vi "Administrators.vi"(11 "数组":string[](array[string])) -> (1 "成功":bool, 2 "子字符串之后":string, 3 "数组 2":string[](array[string]))   [LabVIEW 2018]
panel:
  in  "权限：":string(combo)
  in  "停止":bool
  in  "按钮":bool
  in  "密码：":string
  in  "用户名：":string
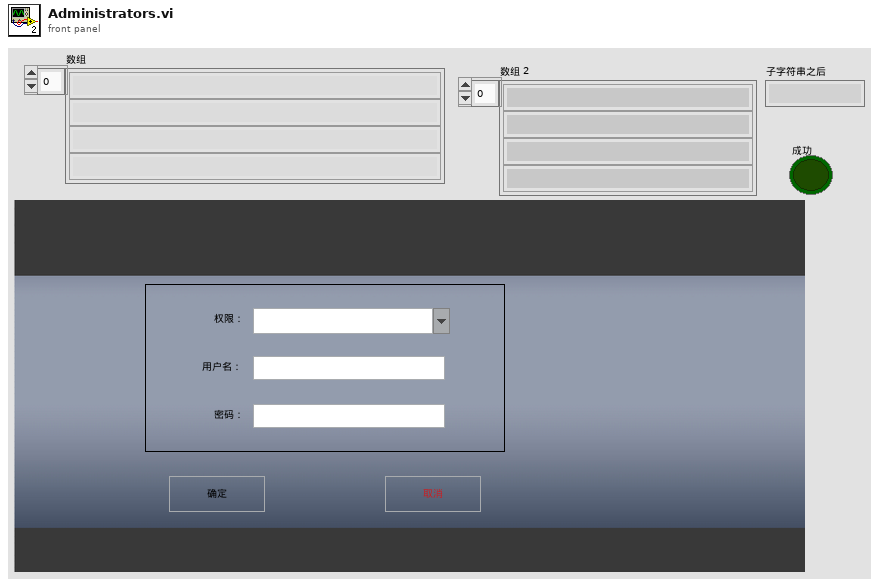
[diagram p1: front panel]
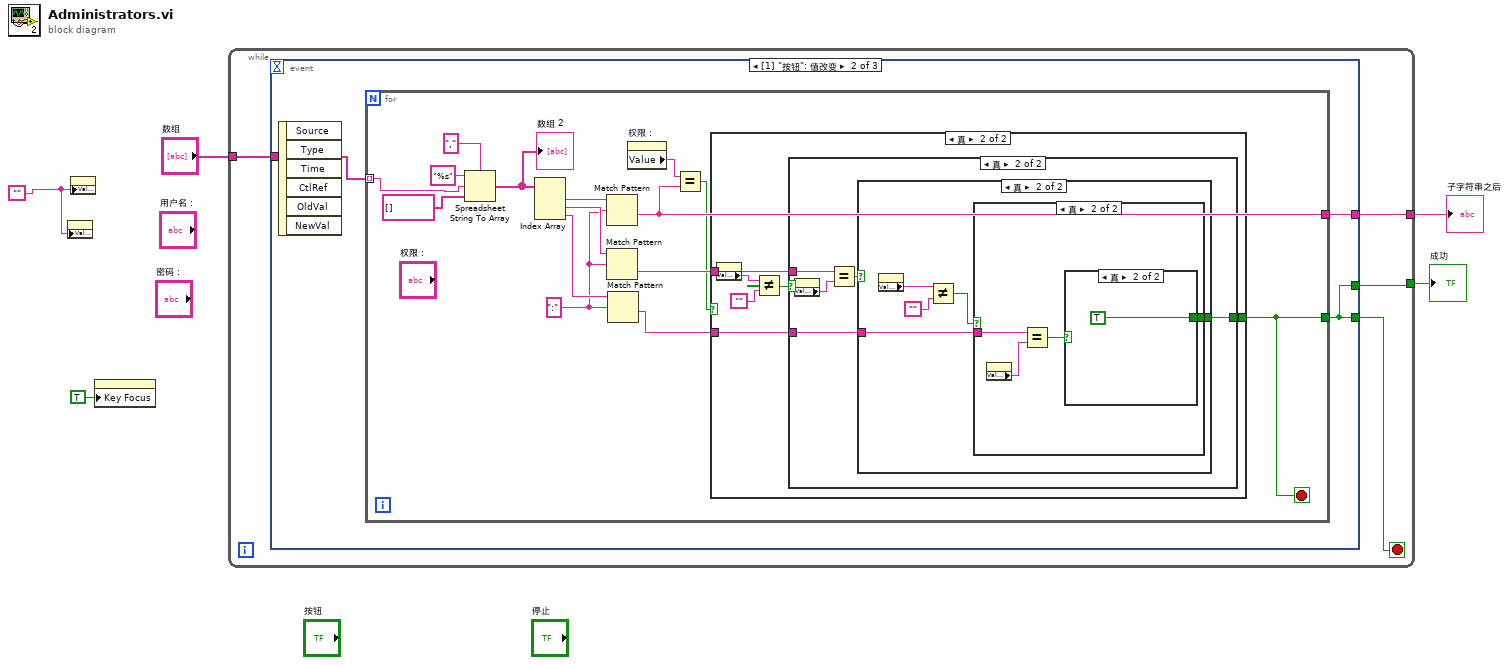
[diagram p0: block diagram]
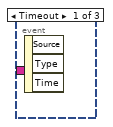
[diagram p2: hidden frame]
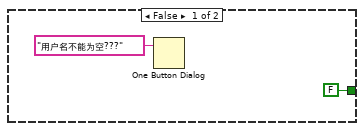
[diagram p4: hidden frame]
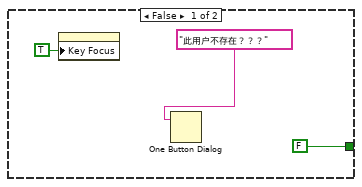
[diagram p5: hidden frame]
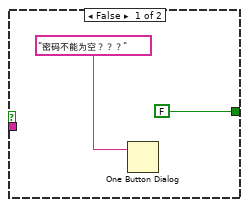
[diagram p6: hidden frame]
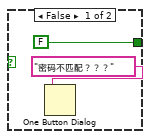
[diagram p7: hidden frame]
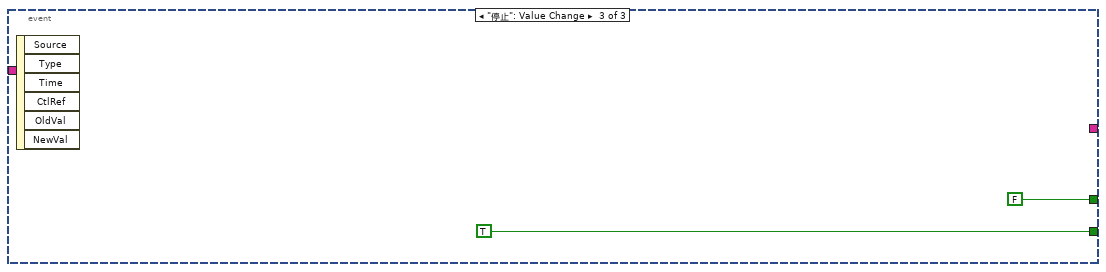
[diagram p8: hidden frame]
diagram:
  w2 = ""
  n1 = property on="密码：" class="Str"("Value"=w2) -> ()  [unwired: 2 in, 2 out]
  n2 = property on="用户名：" class="Str"("Value"=w2) -> ()  [unwired: 2 in, 2 out]
  n3 = property on="用户名：" class="Str"("Key Focus"=TRUE ("键选中")) -> ()  [unwired: 2 in, 2 out]
  n4 = while {
    tunnel: "数组" -> [w9]
    tunnel: [w8] -> w4
    tunnel: [w6] -> w1
    stop <- w7 stop-if-true
    n5 = event shown="[1] \"按钮\": 值改变" {
      selector: _ -> [_ _ _]
      dyn-events: _ -> [_ _ _]
      timeout: _ -> [_ _ _]
      tunnel: w9 -> [_ w12 _]
      tunnel: [_ w10 TRUE] -> w7
      tunnel: [_ w11 _] -> w8
      tunnel: [_ w10 FALSE] -> w6
      event Timeout {
        n6 = event-data() -> ()  [unwired: 1 in, 3 out]
      }
      event "按钮": Value Change {
        n7 = event-data() -> ()  [unwired: 1 in, 6 out]
        n8 = for {
          tunnel: w12 -> [w24] mode=indexing
          tunnel: [w15] -> w11
          tunnel: [w13] -> w10
          stop <- w13 stop-if-true
          w19 = ":" ("正则表达式")
          n9 = Spreadsheet String To Array(delimiter (Tab)="," ("分隔符(Tab)"), format string="%s" ("格式字符串"), spreadsheet string=w24, array type (2D Dbl)=string[] []) -> (array=w23:string[])
          "数组 2" <- w23
          n10 = Index Array(array=w23) -> (element #1=w22:string, element #2=w21:string, element #3=w20:string)  [unwired: 3 in]
          n11 = Match Pattern(string=w22, regular expression=w19) -> (after substring=w15:string)  [unwired: 1 in, 3 out]
          n12 = Match Pattern(string=w21, regular expression=w19) -> (after substring=w18:string)  [unwired: 1 in, 3 out]
          n13 = Match Pattern(string=w20, regular expression=w19) -> (after substring=w17:string)  [unwired: 1 in, 3 out]
          n14 = property on="权限：" class="CmbBox"() -> ("Value"=w16:string)  [unwired: 2 in, 2 out]
          n15 = Equal?(x=w16, y=w15) -> (x = y?=w14:bool)
          n16 = case shown="真" w14 {
            tunnel: w18 -> [_ w32]
            tunnel: w17 -> [_ w30]
            tunnel: [_ w29] -> w13
            frame False {
            }
            frame True {
              n17 = property on="用户名：" class="Str"() -> ("Value"=w28:string)  [unwired: 2 in, 2 out]
              n18 = Not Equal?(x=w28, y="") -> (x != y?=w31:bool)
              n19 = case shown="真" w31 {
                tunnel: w32 -> [_ w38]
                tunnel: w30 -> [_ w37]
                tunnel: [FALSE w36] -> w29
                frame False {
                  n20 = One Button Dialog(message="用户名不能为空???" ("消息")) -> ()  [unwired: 1 in, 1 out]
                }
                frame True {
                  n21 = property on="用户名：" class="Str"() -> ("Value"=w40:string)  [unwired: 2 in, 2 out]
                  n22 = Equal?(x=w38, y=w40) -> (x = y?=w39:bool)
                  n23 = case shown="真" w39 {
                    tunnel: w37 -> [_ w47]
                    tunnel: [FALSE w45] -> w36
                    frame False {
                      n24 = property on="用户名：" class="Str"("Key Focus"=TRUE ("键选中")) -> ()  [unwired: 2 in, 2 out]
                      n25 = One Button Dialog(message="此用户不存在？？？") -> ()  [unwired: 1 in, 1 out]
                    }
                    frame True {
                      n26 = property on="密码：" class="Str"() -> ("Value"=w44:string)  [unwired: 2 in, 2 out]
                      n27 = Not Equal?(x=w44, y="") -> (x != y?=w46:bool)
                      n28 = case shown="真" w46 {
                        tunnel: w47 -> [_ w54]
                        tunnel: [FALSE w51] -> w45
                        frame False {
                          n29 = One Button Dialog(message="密码不能为空？？？") -> ()  [unwired: 1 in, 1 out]
                        }
                        frame True {
                          n30 = property on="密码：" class="Str"() -> ("Value"=w53:string)  [unwired: 2 in, 2 out]
                          n31 = Equal?(x=w54, y=w53) -> (x = y?=w52:bool)
                          n32 = case shown="真" w52 {
                            tunnel: [FALSE TRUE] -> w51
                            frame False {
                              n33 = One Button Dialog(message="密码不匹配？？？") -> ()  [unwired: 1 in, 1 out]
                            }
                            frame True {
                            }
                          }
                        }
                      }
                    }
                  }
                }
              }
            }
          }
        }
      }
      event "停止": Value Change {
        n34 = event-data() -> ()  [unwired: 1 in, 6 out]
      }
    }
  }
  "子字符串之后" <- w4
  "成功" <- w1
